vi "Filter Menu Items.vi"(8 "error in (no error)":errorcluster, 9 "Bit threshold":i32, 11 "flatMenu[] in":T1=[{"menuTag"="", "itemName"="Remove"}, {"menuTag"="", "itemName"="Duplicate"}, {"menuTag"="", "itemName"="Add"}, {"menuTag"="Add", "itemName"="Boolean"}, {"menuTag"="Add", "itemName"="I8"}, {"menuTag"="Add", "itemName"="U8"}, {"menuTag"="Add", "itemName"="I16"}, {"menuTag"="Add", "itemName"="U16"}, {"menuTag"="Add", "itemName"="I32"}, {"menuTag"="Add", "itemName"="U32"}, {"menuTag"="Add", "itemName"="I64"}, {"menuTag"="Add", "itemName"="U64"}, {"menuTag"="Add", "itemName"="FXPI32"}, {"menuTag"="Add", "itemName"="FXPU32"}, {"menuTag"="Add", "itemName"="FXPI64"}, {"menuTag"="Add", "itemName"="FXPU64"}]) -> (0 "error out":errorcluster, 3 "flatMenu[] out":T1)   [LabVIEW 2013, in "Packet.lvclass"]
uses:
  Packet.lvclass
  xCE/_shared/flatMenu.ctl
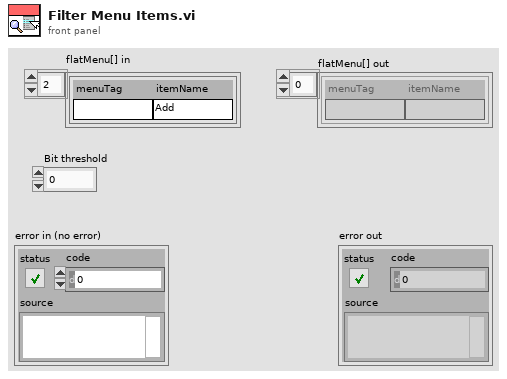
[diagram p1: front panel]
types:
  T1 = typedef "flatMenu.ctl" = cluster{"menuTag":string, "itemName":string}[]
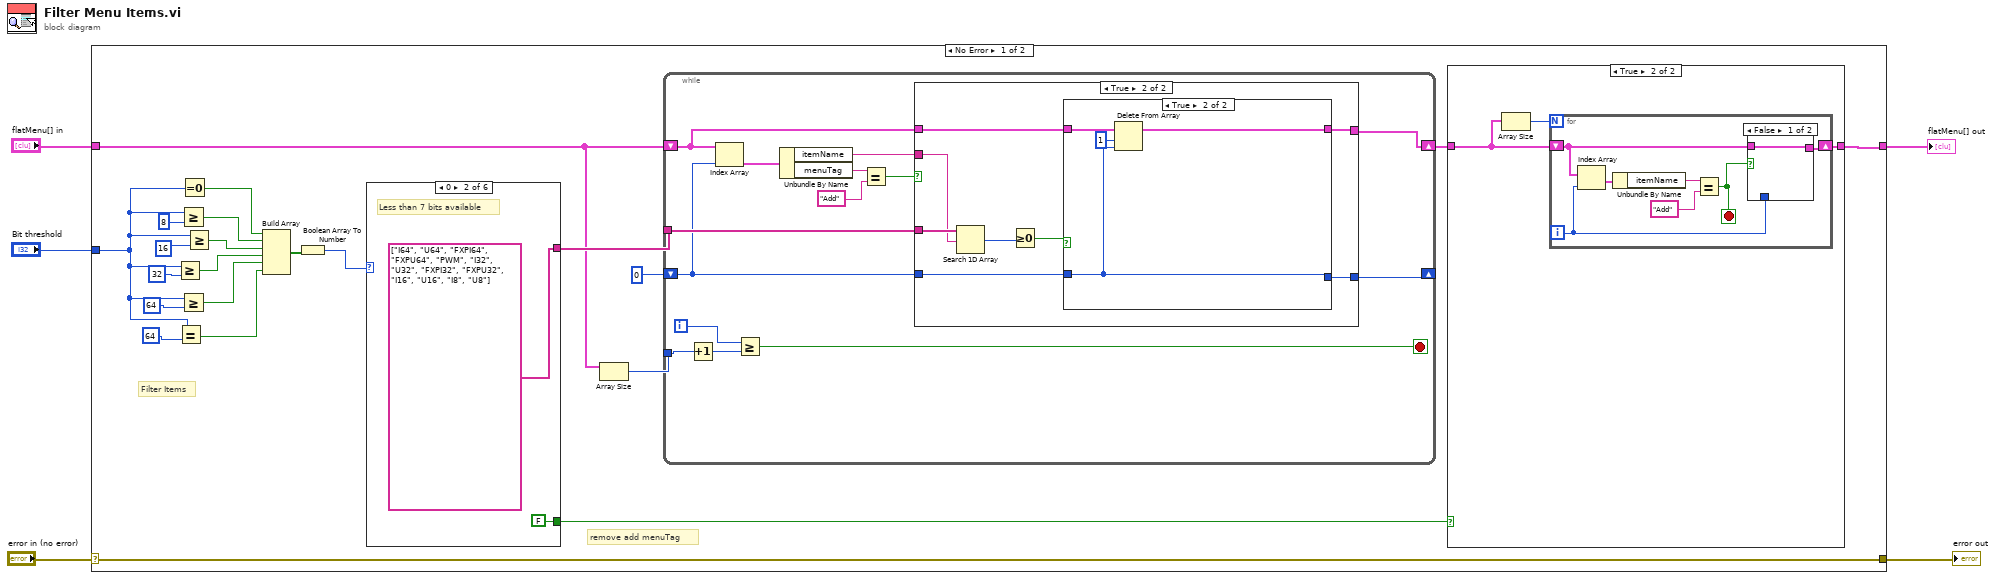
[diagram p0: block diagram]
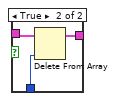
[diagram p3: hidden frame]
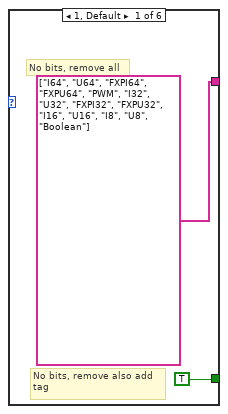
[diagram p4: hidden frame]
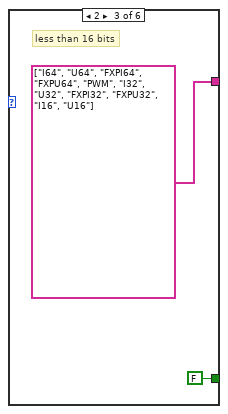
[diagram p5: hidden frame]
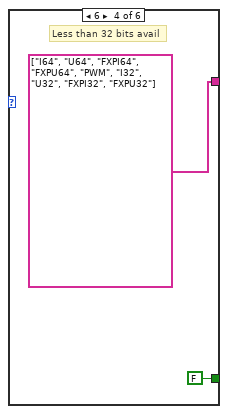
[diagram p6: hidden frame]
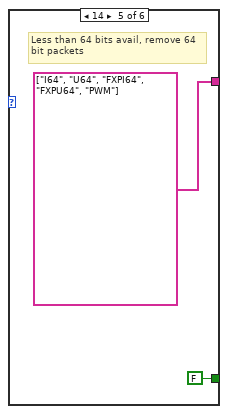
[diagram p7: hidden frame]
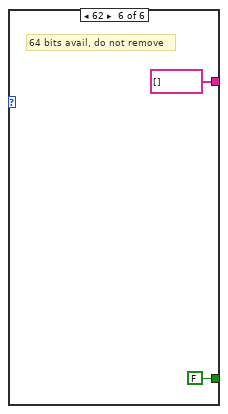
[diagram p8: hidden frame]
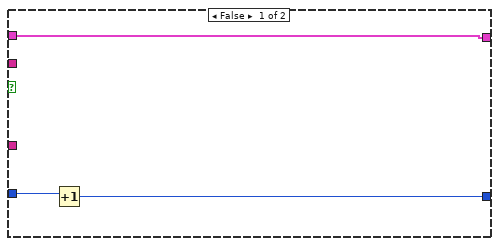
[diagram p9: hidden frame]
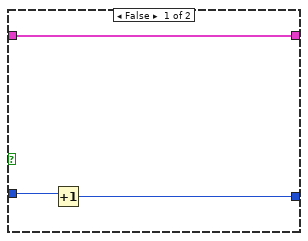
[diagram p10: hidden frame]
diagram:
  n1 = case shown="No Error" "error in (no error)" {
    selector: "error in (no error)" -> [w9 w87]
    tunnel: "flatMenu[] in" -> [w25 w86]
    tunnel: [w7 w86] -> w4
    tunnel: "Bit threshold" -> [w10 _]
    tunnel: [w9 w87] -> w1
    frame No Error {
      # "remove add menuTag"
      # "Filter Items"
      n2 = Greater Or Equal?(x=w10, y=32) -> (x >= y?=w20:bool)
      n3 = Equal?(x=w10, y=64) -> (x = y?=w22:bool)
      n4 = Greater Or Equal?(x=w10, y=8) -> (x >= y?=w18:bool)
      n5 = Greater Or Equal?(x=w10, y=64) -> (x >= y?=w21:bool)
      n6 = Equal To 0?(x=w10) -> (x = 0?=w17:bool)
      n7 = Greater Or Equal?(x=w10, y=16) -> (x >= y?=w19:bool)
      n8 = Build Array(w17, w18, w19, w20, w21, w22) -> (w11:bool[])
      n9 = Boolean Array To Number(Boolean array=w11) -> (number=w27:u32)
      n10 = case shown="0" w27 {
        tunnel: [string[] ["I64", "U64", "FXPI64", "FXPU64", "PWM", "I32", "U32", "FXPI32", "FXPU32", "I16", "U16", "I8", "U8", "Boolean"] string[] ["I64", "U64", "FXPI64", "FXPU64", "PWM", "I32", "U32", "FXPI32", "FXPU32", "I16", "U16", "I8", "U8"] string[] ["I64", "U64", "FXPI64", "FXPU64", "PWM", "I32", "U32", "FXPI32", "FXPU32", "I16", "U16"] string[] ["I64", "U64", "FXPI64", "FXPU64", "PWM", "I32", "U32", "FXPI32", "FXPU32"] string[] ["I64", "U64", "FXPI64", "FXPU64", "PWM"] string[] []] -> w26
        tunnel: [TRUE FALSE FALSE FALSE FALSE FALSE] -> w6
        frame 1, Default {
          # "No bits, remove also add\ntag"
          # "No bits, remove all"
        }
        frame 0 {
          # "Less than 7 bits available"
        }
        frame 2 {
          # "less than 16 bits"
        }
        frame 6 {
          # "Less than 32 bits avail"
        }
        frame 14 {
          # "Less than 64 bits avail, remove 64\nbit packets"
        }
        frame 62 {
          # "64 bits avail, do not remove"
        }
      }
      n11 = Array Size(array=w25) -> (size(s)=w24:i32)
      n12 = while {
        shift-right: [w57] -> w8
        shift-left: w25 -> [w58]
        tunnel: w24 -> [w61]
        shift-right: [w55] -> _
        shift-left: 0 -> [w56]
        tunnel: w26 -> [w67]
        i -> [w62]
        stop <- w60 stop-if-true
        n13 = Increment(x=w61) -> ()  [unwired: 1 out]
        n14 = Index Array(array=w58, index=w56) -> (element=w64:cluster{"menuTag":string, "itemName":string})
        n15 = Greater Or Equal?(x=w62, y=w61) -> (x >= y?=w60:bool)
        n16 = Unbundle By Name(w64) -> ("itemName"=w59:string, "menuTag"=w63:string)
        n17 = Equal?(x=w63, y="Add") -> (x = y?=w65:bool)
        n18 = case shown="True" w65 {
          tunnel: w67 -> [_ w78]
          tunnel: w59 -> [_ w77]
          tunnel: w58 -> [w68 w75]
          tunnel: [w68 w73] -> w57
          tunnel: w56 -> [w70 w72]
          tunnel: [w69 w71] -> w55
          frame False {
            n19 = Increment(x=w70) -> (x+1=w69:i32)
          }
          frame True {
            n20 = Search 1D Array(1D array=w78, element=w77) -> (index of element=w74:i32)  [unwired: 1 in]
            n21 = Greater Or Equal To 0?(x=w74) -> (x >= 0?=w76:bool)
            n22 = case shown="True" w76 {
              tunnel: w75 -> [w81 w85]
              tunnel: [w81 w83] -> w73
              tunnel: w72 -> [w80 w82]
              tunnel: [w79 w82] -> w71
              frame False {
                n23 = Increment(x=w80) -> (x+1=w79:i32)
              }
              frame True {
                n24 = Delete From Array(array=w85, length=1, index=w82) -> (array with subset deleted=w83:T1)  [unwired: 1 out]
              }
            }
          }
        }
      }
      n25 = case shown="True" w6 {
        tunnel: w8 -> [w28 w30]
        tunnel: [w28 w31] -> w7
        frame False {
        }
        frame True {
          n26 = Array Size(array=w30) -> (size(s)=w29:i32)
          n27 = for {
            N: w29 -> [_]
            shift-right: [w32] -> w31
            shift-left: w30 -> [w34]
            i -> [w33]
            stop <- w35 stop-if-true
            n28 = Index Array(array=w34, index=w33) -> (element=w36:cluster{"menuTag":string, "itemName":string})
            n29 = Unbundle By Name(w36) -> ("itemName"=w38:string)
            n30 = Equal?(x=w38, y="Add") -> (x = y?=w35:bool)
            n31 = case shown="False" w35 {
              tunnel: w34 -> [w39 w42]
              tunnel: w33 -> [_ w41]
              tunnel: [w39 w40] -> w32
              frame False {
              }
              frame True {
                n32 = Delete From Array(array=w42, index=w41) -> (array with subset deleted=w40:T1)  [unwired: 1 in, 1 out]
              }
            }
          }
        }
      }
    }
    frame Error {
    }
  }
  "flatMenu[] out" <- w4
  "error out" <- w1
